vi "Histogram1003.vi"   [LabVIEW 2013]
uses:
  <vilib>/Heliosphere Research LLC/Advanced Plotting Toolkit/api_plotting/Histogram_Automatic.vi
  <vilib>/Heliosphere Research LLC/Advanced Plotting Toolkit/Advanced Plotting Toolkit.lvlib
types:
  T1 = typedef "Advanced Plotting Toolkit.lvlib/PlotID.ctl" = i32
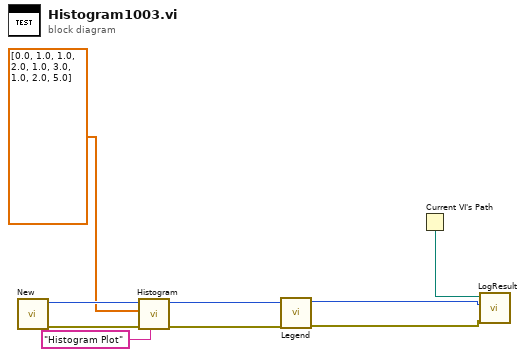
[diagram p0: block diagram]
diagram:
  n1 = call <vilib>:"New.vi"() -> ("error out"=w7:errorcluster, "Plot ID"=w9:T1)  [unwired: 10 in]
  n2 = call-poly <vilib>:"Histogram.vi"("Legend Title"="Histogram Plot", "error in (no error)"=w7, "Data"=dbl[] [0.0, 1.0, 1.0, 2.0, 1.0, 3.0, 1.0, 2.0, 5.0], "Plot ID"=w9) -> ("error out"=w2:errorcluster, "Plot ID Out"=w4:T1)  [unwired: 6 in]
  n3 = call <vilib>:"Legend.vi"("error in (no error)"=w2, "Plot ID"=w4) -> ("error out"=w1:errorcluster, "Plot ID Out"=w3:T1)  [unwired: 8 in]
  n4 = Current VI's Path() -> (path=w8:path)
  n5 = call "LogResult.vi"("Test Result"=w1, "Test Artifact"=w3, "VI Path"=w8) -> ()  [unwired: 9 in]
